vi "Read File scan.vi"(0 "Refnum in":T1, 9 "section names":string[](array[string]), 11 "error in (no error)":errorcluster) -> (2 "scan/command":string, 4 "States Out":string, 6 "bin numbers":cluster{"Bin #s":i32[]}[](array[cluster]), 8 "first scan cmd":string, 15 "error out":errorcluster)   [LabVIEW 2020]
uses:
  <vilib>/Utility/config.llb/Config Data RefNum.ctl
  <vilib>/Utility/config.llb/Read Key (String).vi
  <vilib>/regexp/Match Regular Expression.xnode
  <vilib>/Utility/config.llb/NI_LVConfig.lvlib
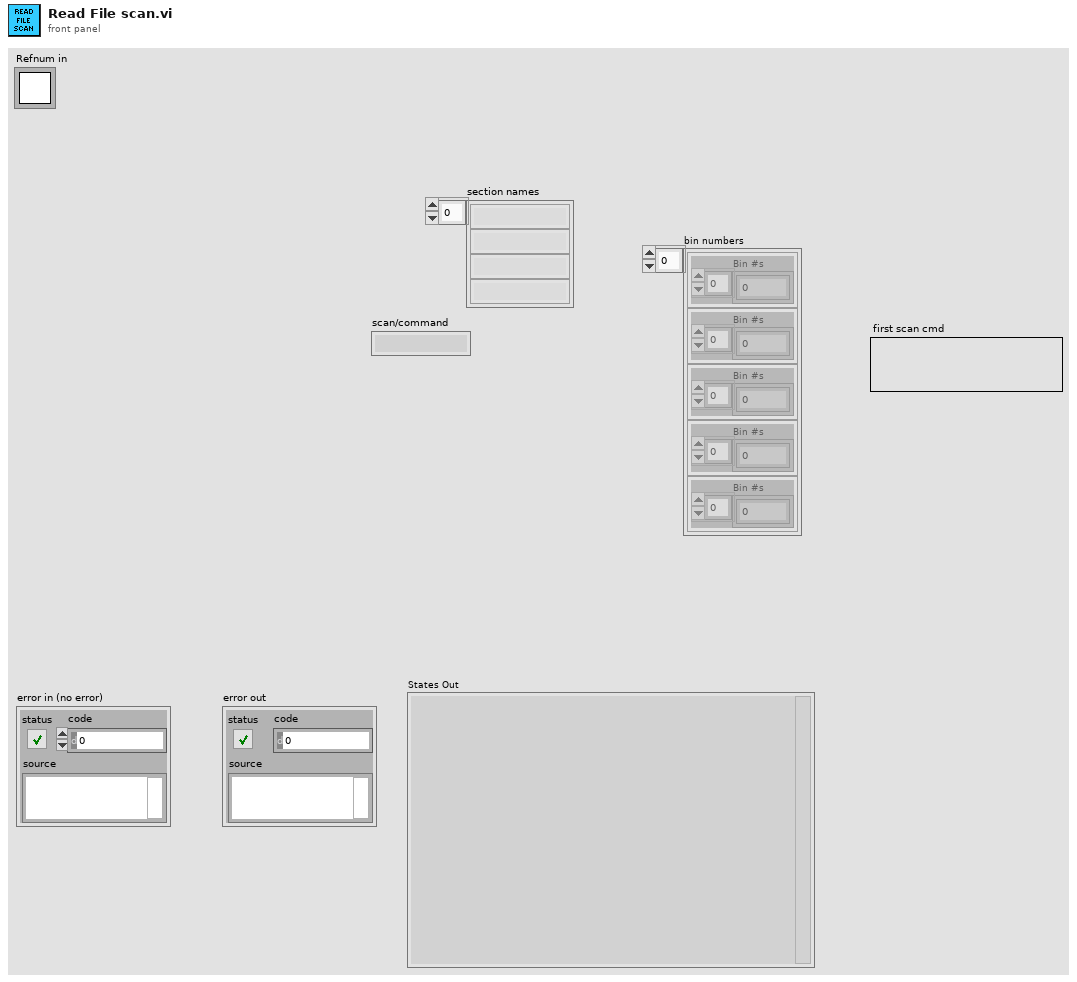
[diagram p1: front panel]
types:
  T1 = typedef "NI_LVConfig.lvlib/Config Data RefNum.ctl" = refnum<k1>
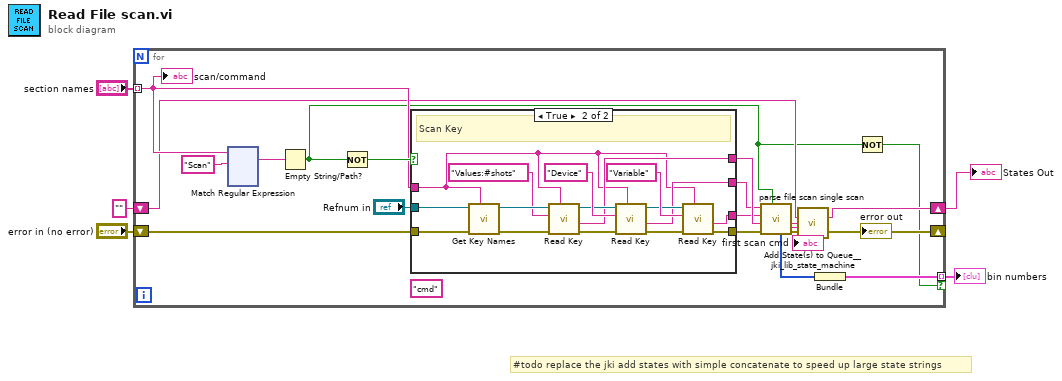
[diagram p0: block diagram]
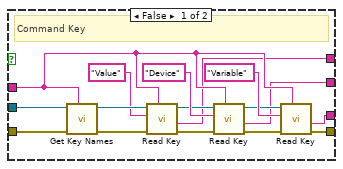
[diagram p2: hidden frame]
diagram:
  # "#todo replace the jki add states with simple concatenate to speed up large state strings"
  n1 = for {
    tunnel: "section names" -> [w16] mode=indexing
    shift-right: [w17] -> w5
    shift-left: "error in (no error)" -> [w15]
    shift-right: [w12] -> w3
    shift-left: "" ("States Out") -> [w14]
    tunnel: [w9] -> w1 mode=indexing if=w7
    (unwired) "cmd" ("Scan/Command")
    n2 = xnode "Match Regular Expression"("input string"=w16, "regular expression"="Scan") -> ("whole match"=w21:string)  [unwired: 4 in, 4 out]
    n3 = Empty String/Path?(string/path=w21) -> (empty?=w8:bool)
    n4 = Not(x=w8) -> (.not. x?=w22:bool)
    n5 = case shown="True" w22 {
      tunnel: "Refnum in" -> [w31 w57]
      tunnel: w15 -> [w32 w56]
      tunnel: [w26 w46] -> w18
      tunnel: [w28 w45] -> w24
      tunnel: [w27 w44] -> w23
      tunnel: [w29 w43] -> w25
      tunnel: w16 -> [w30 w42]
      frame False {
        # "Command Key"
        n6 = call <vilib>:"Get Key Names.vi"("section"=w30, "error in (no error)"=w32, "refnum"=w31) -> ("error out"=w40:errorcluster, "refnum out"=w41:T1)  [unwired: 5 in, 2 out]
        n7 = call-poly <vilib>:"Read Key.vi"("section"=w30, "error in (no error)"=w40, "key"="Value" ("section"), "refnum"=w41) -> ("error out"=w34:errorcluster, "value"=w29:string, "refnum out"=w37:T1)  [unwired: 4 in, 1 out]
        n8 = call-poly <vilib>:"Read Key.vi"("section"=w30, "error in (no error)"=w34, "key"="Device", "refnum"=w37) -> ("error out"=w33:errorcluster, "value"=w28:string, "refnum out"=w35:T1)  [unwired: 4 in, 1 out]
        n9 = call-poly <vilib>:"Read Key.vi"("section"=w30, "error in (no error)"=w33, "key"="Variable", "refnum"=w35) -> ("error out"=w26:errorcluster, "value"=w27:string)  [unwired: 4 in, 2 out]
      }
      frame True {
        # "Scan Key"
        n10 = call <vilib>:"Get Key Names.vi"("section"=w42, "error in (no error)"=w56, "refnum"=w57) -> ("error out"=w54:errorcluster, "refnum out"=w55:T1)  [unwired: 5 in, 2 out]
        n11 = call-poly <vilib>:"Read Key.vi"("section"=w42, "error in (no error)"=w54, "key"="Values:#shots" ("section"), "refnum"=w55) -> ("error out"=w48:errorcluster, "value"=w43:string, "refnum out"=w51:T1)  [unwired: 4 in, 1 out]
        n12 = call-poly <vilib>:"Read Key.vi"("section"=w42, "error in (no error)"=w48, "key"="Device", "refnum"=w51) -> ("error out"=w47:errorcluster, "value"=w45:string, "refnum out"=w49:T1)  [unwired: 4 in, 1 out]
        n13 = call-poly <vilib>:"Read Key.vi"("section"=w42, "error in (no error)"=w47, "key"="Variable", "refnum"=w49) -> ("error out"=w46:errorcluster, "value"=w44:string)  [unwired: 4 in, 2 out]
      }
    }
    n14 = call "parse file scan single scan.vi"("command"=w8, "error in (no error)"=w18, "values and # shots"=w25, "variables"=w23, "Devices"=w24) -> ("error out"=w17:errorcluster, "States Out"=w13:string, "Bin #s"=w10:i32[], "first scan cmd"=→"first scan cmd":string)  [unwired: 3 out]
    n15 = call <vilib>:"Add State(s) to Queue__jki_lib_state_machine.vi"("State(s) in (\"\")"=w14, "State(s) at Back (\"\")"=w13) -> ("States Out"=w12:string)  [unwired: 13 in]
    n16 = Bundle("Bin #s"=w10) -> (w9:cluster{"Bin #s":i32[]})  [unwired: 1 in]
    n17 = Not(x=w8) -> (.not. x?=w7:bool)
    "scan/command" <- w16
  }
  "error out" <- w5
  "States Out" <- w3
  "bin numbers" <- w1
